vi "get gain.vi"(8 "error in (no error)":errorcluster, 11 "Thorcam in":refnum<class "Thorcam.lvclass">) -> (0 "error out":errorcluster, 3 "Thorcam out":refnum<class "Thorcam.lvclass">)   [LabVIEW 2012, in "Thorcam.lvclass"]
uses:
  Thorcam.lvclass
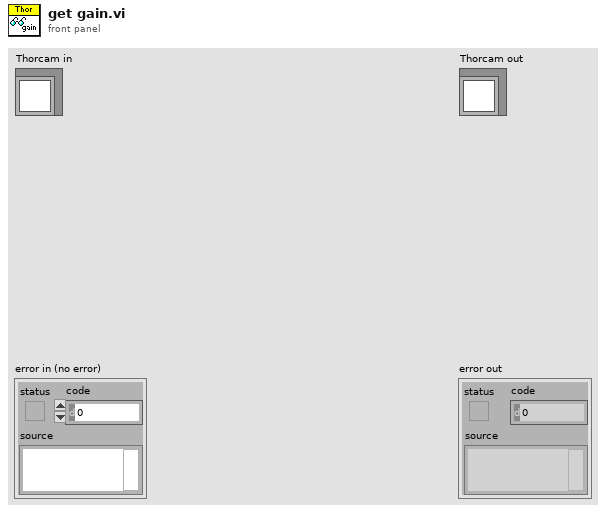
[diagram p1: front panel]
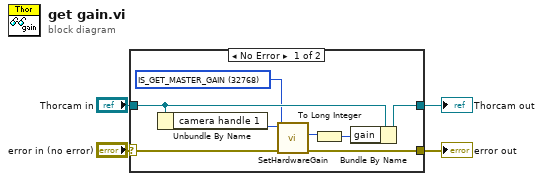
[diagram p0: block diagram]
diagram:
  n1 = case shown="No Error" "error in (no error)" {
    selector: "error in (no error)" -> [w9 w14]
    tunnel: [w8 w14] -> w3
    tunnel: [w11 w13] -> w1
    tunnel: "Thorcam in" -> [w12 w13]
    frame No Error {
      w5 = 32768 items=["IS_GET_MASTER_GAIN"=32768, "IS_GET_RED_GAIN"=32769, "IS_GET_GREEN_GAIN"=32770, "IS_GET_BLUE_GAIN"=32771, "IS_GET_DEFAULT_MASTER"=32772, "IS_GET_DEFAULT_RED"=32773, "IS_GET_DEFAULT_GREEN"=32774, "IS_GET_DEFAULT_BLUE"=32775, "IS_SET_GAIN"=34816] ("Mode")
      n2 = Unbundle By Name(w12) -> ("camera handle 1"=w10:u32)
      n3 = call <instrlib>:"SetHardwareGain.vi"("error in"=w9, "Mode"=w5, "Camera Handle In"=w10) -> ("error out"=w8:errorcluster, "Value"=w7:i32)  [unwired: 6 in, 1 out]
      n4 = To Long Integer(number=w7) -> (32bit integer=w6:i32)
      n5 = Bundle By Name(cluster=w12, "gain"=w6) -> (w11:refnum<class "Thorcam.lvclass">)
    }
    frame Error {
    }
  }
  "error out" <- w3
  "Thorcam out" <- w1
